vi "Variant to Variant Array.vi"(8 "error in (no error)":errorcluster, 11 "value":variant) -> (0 "error out":errorcluster, 3 "Variant (1D array)":variant[](array[variant]))   [LabVIEW 2019, in "Control Experiment.lvclass"]
uses:
  Control Experiment.lvclass
  <vilib>/Utility/Data Type/NI_Data Type.lvlib
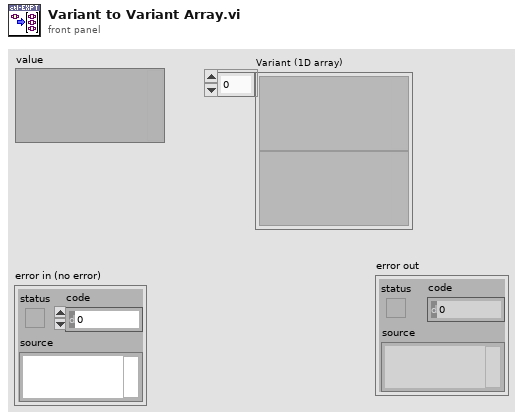
[diagram p1: front panel]
types:
  T1 = typedef "NI_Data Type.lvlib/Data Type.ctl" = enum8{"Invalid Type", "Void", "I8", "I16", "I32", "I64", "U8", "U16", "U32", "U64", "Single Float", "Double Float", "Extended Float", "Single Complex", "Double Complex", "Extended Complex", "Enum U8", "Enum U16", "Enum U32", "Enum U64", "Single Float With Unit", "Double Float With Unit", "Extended Float With Unit", "Single Complex with Unit", "Double Complex with Unit", "Extended Complex with Unit", "Boolean", "String", "Path", "Picture", "Tag", "Array", "Cluster", "Variant", "LV Variant", "Waveform", "Timestamp", "Digital Waveform", "Digital Data", "ExpressData", "Refnum", "External Data", "VI", "Poly VI", "LabVIEW Class Instance", "Fixed Point", "Set Collection", "Map Collection"}
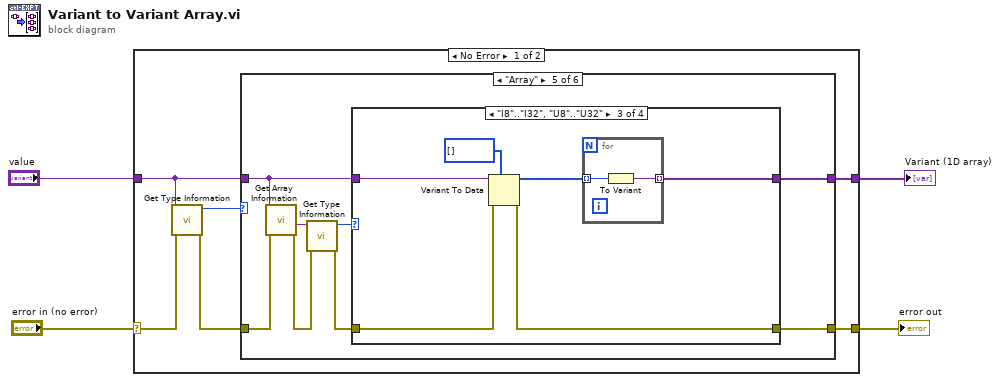
[diagram p0: block diagram]
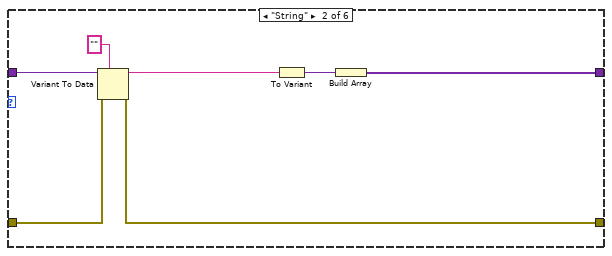
[diagram p3: hidden frame]
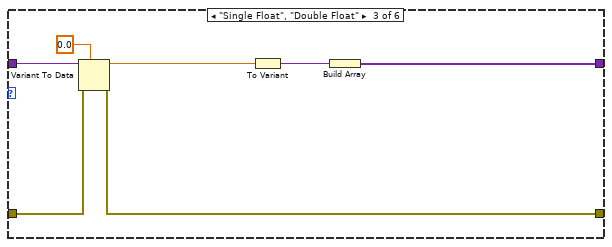
[diagram p4: hidden frame]
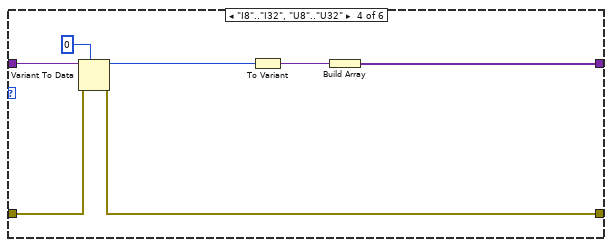
[diagram p5: hidden frame]
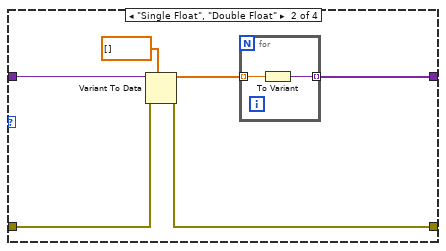
[diagram p7: hidden frame]
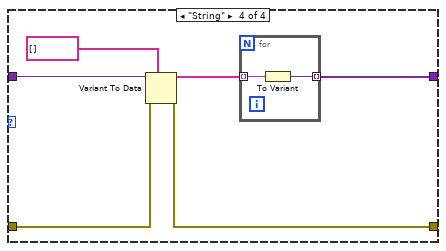
[diagram p8: hidden frame]
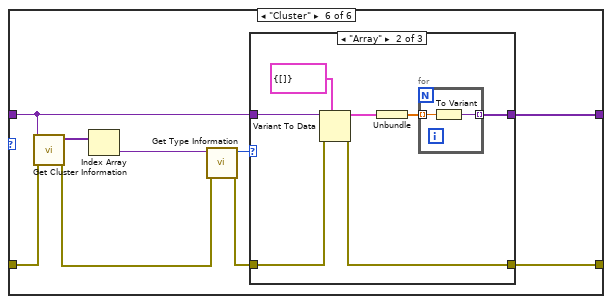
[diagram p9: hidden frame]
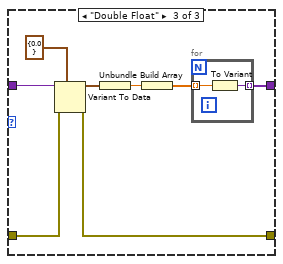
[diagram p11: hidden frame]
diagram:
  n1 = case shown="No Error" "error in (no error)" {
    selector: "error in (no error)" -> [w7 w95]
    tunnel: [w8 w95] -> w3
    tunnel: "value" -> [w5 _]
    tunnel: [w9 _] -> w1
    frame No Error {
      n2 = call <vilib>:"Get Type Information.vi"("error in (no error)"=w7, "variant"=w5) -> ("error out"=w6:errorcluster, "type"=w10:T1)  [unwired: 5 in, 3 out]
      n3 = case shown="\"Array\"" w10 {
        tunnel: [_ w12 w19 w26 w39 w69] -> w9
        tunnel: w5 -> [_ w17 w25 w32 w38 w67]
        tunnel: w6 -> [w11 w15 w24 w31 w37 w74]
        tunnel: [w11 w16 w22 w29 w40 w68] -> w8
        frame Default {
        }
        frame "String" {
          n4 = Variant To Data(error in=w15, type="", Variant=w17) -> (data=w14:string, error out=w16:errorcluster)
          n5 = To Variant(anything=w14) -> (Variant=w13:variant)
          n6 = Build Array(w13) -> (w12:variant[])
        }
        frame "Single Float", "Double Float" {
          n7 = Variant To Data(error in=w24, type=0.0, Variant=w25) -> (data=w21:dbl, error out=w22:errorcluster)
          n8 = To Variant(anything=w21) -> (Variant=w20:variant)
          n9 = Build Array(w20) -> (w19:variant[])
        }
        frame "I8".."I32", "U8".."U32" {
          n10 = Variant To Data(error in=w31, type=0, Variant=w32) -> (data=w28:i32, error out=w29:errorcluster)
          n11 = To Variant(anything=w28) -> (Variant=w27:variant)
          n12 = Build Array(w27) -> (w26:variant[])
        }
        frame "Array" {
          n13 = call <vilib>:"Get Array Information.vi"("error in (no error)"=w37, "variant"=w38) -> ("error out"=w34:errorcluster, "array element data type"=w36:variant)  [unwired: 6 in, 2 out]
          n14 = call <vilib>:"Get Type Information.vi"("error in (no error)"=w34, "variant"=w36) -> ("error out"=w33:errorcluster, "type"=w35:T1)  [unwired: 5 in, 3 out]
          n15 = case shown="\"I8\"..\"I32\", \"U8\"..\"U32\"" w35 {
            tunnel: [w41 w46 w54 w62] -> w40
            tunnel: [_ w42 w50 w60] -> w39
            tunnel: w38 -> [_ w44 w52 w59]
            tunnel: w33 -> [w41 w43 w51 w58]
            frame Default {
            }
            frame "Single Float", "Double Float" {
              n16 = Variant To Data(error in=w43, type=dbl[] [], Variant=w44) -> (data=w45:dbl[], error out=w46:errorcluster)
              n17 = for {
                tunnel: w45 -> [w49] mode=indexing
                tunnel: [w48] -> w42 mode=indexing
                n18 = To Variant(anything=w49) -> (Variant=w48:variant)
              }
            }
            frame "I8".."I32", "U8".."U32" {
              n19 = Variant To Data(error in=w51, type=i32[] [], Variant=w52) -> (data=w53:i32[], error out=w54:errorcluster)
              n20 = for {
                tunnel: w53 -> [w57] mode=indexing
                tunnel: [w56] -> w50 mode=indexing
                n21 = To Variant(anything=w57) -> (Variant=w56:variant)
              }
            }
            frame "String" {
              n22 = Variant To Data(error in=w58, type=string[] [], Variant=w59) -> (data=w61:string[], error out=w62:errorcluster)
              n23 = for {
                tunnel: w61 -> [w65] mode=indexing
                tunnel: [w64] -> w60 mode=indexing
                n24 = To Variant(anything=w65) -> (Variant=w64:variant)
              }
            }
          }
        }
        frame "Cluster" {
          n25 = call <vilib>:"Get Cluster Information.vi"("error in (no error)"=w74, "variant"=w67) -> ("error out"=w72:errorcluster, "cluster elements"=w73:variant[])  [unwired: 8 in]
          n26 = Index Array(array=w73) -> (element=w71:variant)  [unwired: 1 in]
          n27 = call <vilib>:"Get Type Information.vi"("error in (no error)"=w72, "variant"=w71) -> ("error out"=w66:errorcluster, "type"=w70:T1)  [unwired: 5 in, 3 out]
          n28 = case shown="\"Array\"" w70 {
            tunnel: [_ w77 w85] -> w69
            tunnel: w67 -> [_ w81 w91]
            tunnel: w66 -> [w75 w80 w90]
            tunnel: [w75 w76 w88] -> w68
            frame Default {
            }
            frame "Array" {
              n29 = Variant To Data(error in=w80, type=cluster{dbl[]} {[]}, Variant=w81) -> (data=w82:cluster{dbl[]}, error out=w76:errorcluster)
              n30 = Unbundle(w82) -> (w78:dbl[])
              n31 = for {
                tunnel: w78 -> [w84] mode=indexing
                tunnel: [w83] -> w77 mode=indexing
                n32 = To Variant(anything=w84) -> (Variant=w83:variant)
              }
            }
            frame "Double Float" {
              n33 = Variant To Data(error in=w90, type=cluster{dbl} {0.0}, Variant=w91) -> (data=w92:cluster{dbl}, error out=w88:errorcluster)
              n34 = Unbundle(w92) -> (w86:dbl)
              n35 = Build Array(w86) -> (w89:dbl[])
              n36 = for {
                tunnel: w89 -> [w94] mode=indexing
                tunnel: [w93] -> w85 mode=indexing
                n37 = To Variant(anything=w94) -> (Variant=w93:variant)
              }
            }
          }
        }
      }
    }
    frame Error {
    }
  }
  "error out" <- w3
  "Variant (1D array)" <- w1
